vi "Configure Transfer Groups.vi"(8 "error in (no error)":errorcluster, 10 "Transfer Groups":refnum<class "Transfer Group.lvclass">[](array[class]), 11 "Plugin in":refnum<class "Plugin.lvclass">) -> (0 "error out":errorcluster, 3 "Plugin out":refnum<class "Plugin.lvclass">)   [LabVIEW 2017, in "DSF Core.lvlib" / "Plugin.lvclass"]
uses:
  Plugin.lvclass
  Transfer Group/Transfer Group.lvclass
  Plugin.lvclass/Plugin.ctl
  Timing/Timing.lvclass
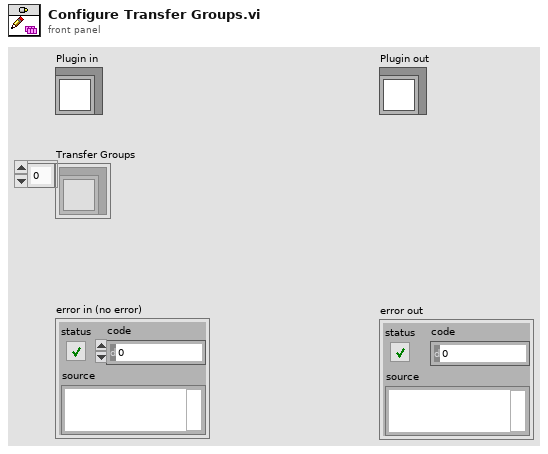
[diagram p1: front panel]
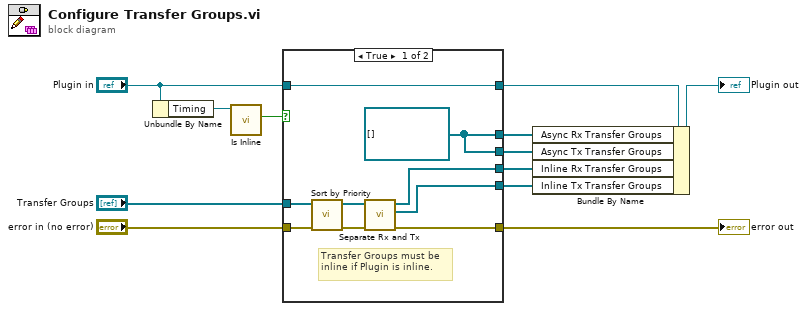
[diagram p0: block diagram]
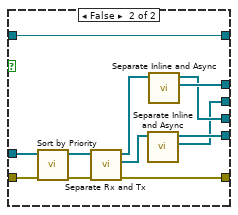
[diagram p2: hidden frame]
diagram:
  n1 = Unbundle By Name("Plugin in") -> ("Timing"=w8:refnum<class "Timing.lvclass">)
  n2 = call "Is Inline.vi"("Timing in"=w8) -> ("inline?"=w1:bool)  [unwired: 9 in, 1 out]
  n3 = case shown="True" w1 {
    tunnel: "Plugin in" -> [w13 w33]
    tunnel: [w13 w33] -> w11
    tunnel: "Transfer Groups" -> [w21 w32]
    tunnel: "error in (no error)" -> [w18 w29]
    tunnel: [w17 w24] -> w12
    tunnel: [w16 w25] -> w6
    tunnel: [w15 w23] -> w5
    tunnel: [w14 w22] -> w4
    tunnel: [w14 w26] -> w7
    frame True {
      w14 = refnum<class "Transfer Group.lvclass">[] [] ("Async Transfer Groups")
      # "Transfer Groups must be inline if Plugin is inline."
      n4 = call "Sort by Priority.vi"("error in (no error)"=w18, "Transfer Groups"=w21) -> ("error out"=w19:errorcluster, "sorted Transfer Groups"=w20:refnum<class "Transfer Group.lvclass">[])  [unwired: 8 in]
      n5 = call "Separate Rx and Tx.vi"("error in (no error)"=w19, "Transfer Groups"=w20) -> ("error out"=w17:errorcluster, "Tx Transfer Groups"=w16:refnum<class "Transfer Group.lvclass">[], "Rx Transfer Groups"=w15:refnum<class "Transfer Group.lvclass">[])  [unwired: 7 in]
    }
    frame False {
      n6 = call "Sort by Priority.vi"("error in (no error)"=w29, "Transfer Groups"=w32) -> ("error out"=w30:errorcluster, "sorted Transfer Groups"=w31:refnum<class "Transfer Group.lvclass">[])  [unwired: 8 in]
      n7 = call "Separate Rx and Tx.vi"("error in (no error)"=w30, "Transfer Groups"=w31) -> ("error out"=w24:errorcluster, "Tx Transfer Groups"=w27:refnum<class "Transfer Group.lvclass">[], "Rx Transfer Groups"=w28:refnum<class "Transfer Group.lvclass">[])  [unwired: 7 in]
      n8 = call "Separate Inline and Async.vi"("Transfer Groups"=w27) -> ("Async Transfer Groups"=w22:refnum<class "Transfer Group.lvclass">[], "Inline Transfer Groups"=w25:refnum<class "Transfer Group.lvclass">[])  [unwired: 8 in, 1 out]
      n9 = call "Separate Inline and Async.vi"("Transfer Groups"=w28) -> ("Async Transfer Groups"=w26:refnum<class "Transfer Group.lvclass">[], "Inline Transfer Groups"=w23:refnum<class "Transfer Group.lvclass">[])  [unwired: 8 in, 1 out]
    }
  }
  "error out" <- w12
  n10 = Bundle By Name(cluster=w11, "Async Rx Transfer Groups"=w7, "Async Tx Transfer Groups"=w4, "Inline Rx Transfer Groups"=w5, "Inline Tx Transfer Groups"=w6) -> (→"Plugin out":refnum<class "Plugin.lvclass">)
